vi "New.vi"(6 "rect in":T1, 7 "picture":picture, 9 "Radius in":i16, 10 "color in":u32(colorbox)) -> (3 "Goal post out":refnum<class "Goal Post.lvclass">, 5 "picture out":picture)   [LabVIEW 2024, in "Goal Post.lvclass"]
doc: "MIT Licence\nCopyright (c) 2024 David Grollier"
uses:
  Goal Post.lvclass
  Type Def/Coordinates.ctl
  Goal Post.lvclass/Goal Post.ctl
  Game Componants.lvclass/Game Componants.ctl
  Game Componants.lvclass
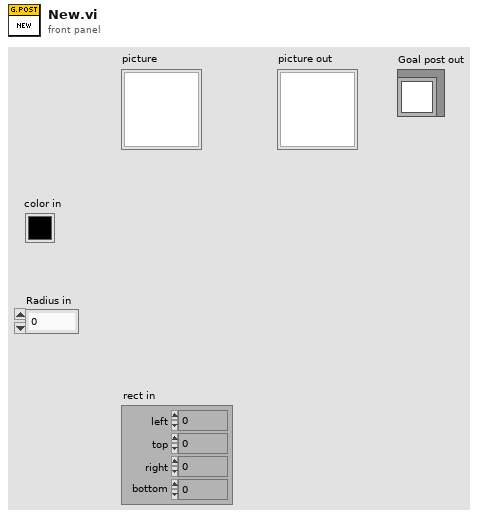
[diagram p1: front panel]
types:
  T1 = cluster{"left":i16, "top":i16, "right":i16, "bottom":i16}
  T2 = typedef "Coordinates.ctl" = cluster{"x":dbl, "y":dbl}
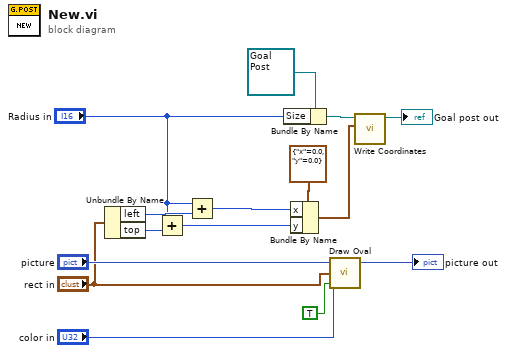
[diagram p0: block diagram]
diagram:
  n1 = Unbundle By Name("rect in") -> ("left"=w8:i16, "top"=w3:i16)
  n2 = Add(x="Radius in", y=w3) -> (x+y=w1:i16)
  n3 = Add(x="Radius in", y=w8) -> (x+y=w4:i16)
  n4 = Bundle By Name(cluster=refnum<class "Goal Post.lvclass"> refnum ("Goal post in"), "Size"="Radius in") -> (w7:refnum<class "Goal Post.lvclass">)
  n5 = Bundle By Name(cluster=T2 {"x"=0.0, "y"=0.0} ("Coordinates"), "x"=w4, "y"=w1) -> (w5:T2)
  n6 = call <vilib>:"Draw Oval.vi"("picture"="picture", "rect"="rect in", "fill?(F)"=TRUE, "color(black)"="color in") -> ("new picture"=→"picture out":picture)  [unwired: 5 in]
  n7 = call "Write Coordinates.vi"("Coordinates"=w5, "Game Componants in"=w7) -> ("Game Componants out"=→"Goal post out":refnum<class "Goal Post.lvclass">)  [unwired: 9 in]
